vi "动态信号.vi"() -> ()   [LabVIEW 2018]
uses:
  <vilib>/express/express shared/transition.llb/Dynamic To Waveform Array.vi
  <vilib>/express/express signal manip/GetorSetDDTAttributes/Get DDT Attributes/Get DDT Properties.xnode
panel:
  out "单位":string
  out "时间标识":timestamp
  out "信号名称":string
  out "Array of Waveform":waveform(dbl)[](array[waveform]) caption="波形数组"
  out "正弦":dynamicdata(graph)
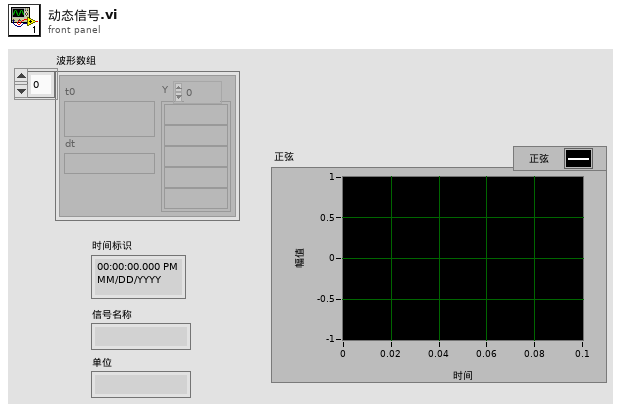
[diagram p1: front panel]
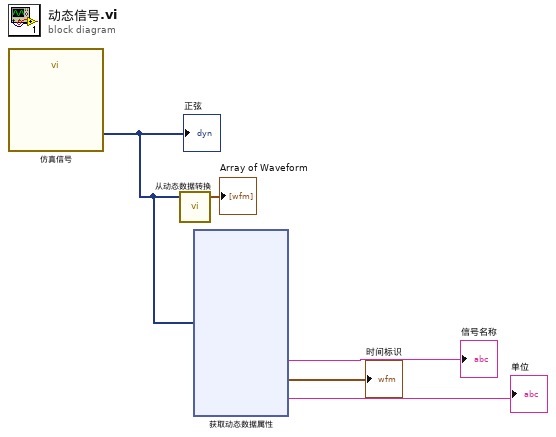
[diagram p0: block diagram]
diagram:
  n1 = call "仿真信号"() -> ("正弦"=w4:dynamicdata)  [unwired: 14 in, 1 out]
  "正弦" <- w4
  n2 = call "从动态数据转换"("Dynamic Data Type"=w4) -> ("Array of Waveform"=→"Array of Waveform":waveform(dbl)[])  [unwired: 3 in]
  n3 = xnode "获取动态数据属性"("信号输入"=w4) -> ("信号名称"=→"信号名称":string, "时间标识"=→"时间标识":timestamp, "单位"=→"单位":string)  [unwired: 2 in, 2 out]
